vi "phone database.vi"() -> ()   [LabVIEW 2011]
uses:
  <vilib>/addons/database/Auxilliary.llb/DB Tools DataTypes.ctl
  <vilib>/addons/database/Connection.llb/DB Tools Open Connec (Path).vi
  <vilib>/addons/database/NI_Database_API.lvlib
panel:
  out "data":variant[][](array[variant])
  out "column information":T2(array[cluster])
  out "columns":string[](array[string])
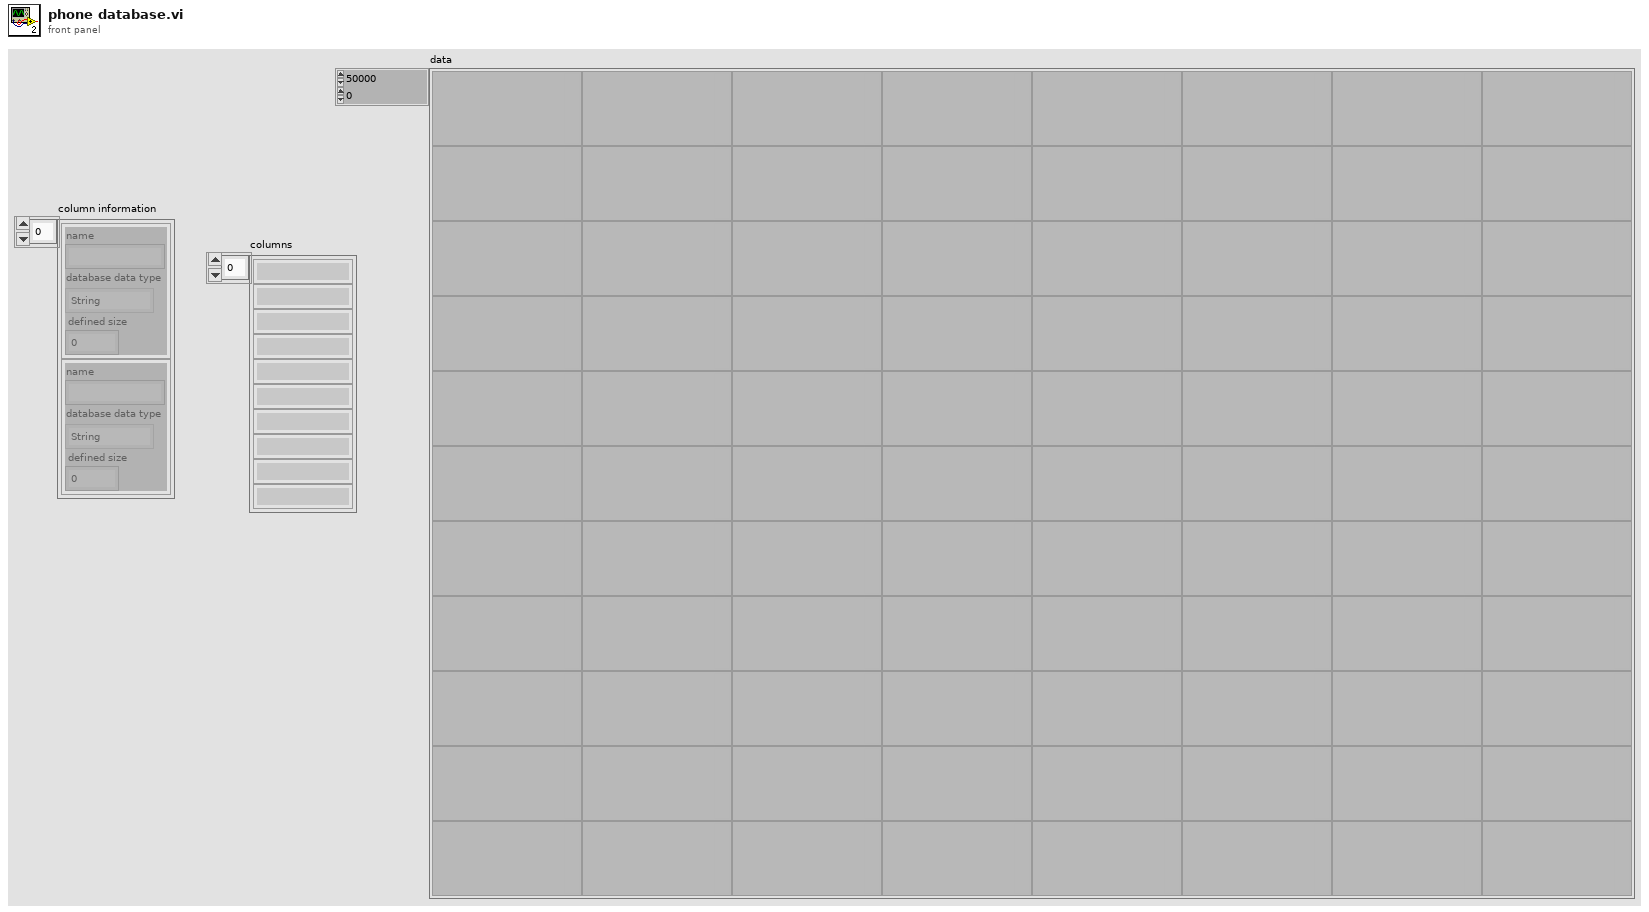
[diagram p1: front panel]
types:
  T1 = typedef "NI_Database_API.lvlib/DB Tools DataTypes.ctl" = enum16{"String", "Long (I32)", "Single (SGL)", "Double (DBL)", "Date/Time", "Binary"}
  T2 = cluster{"name":string, "database data type":T1, "defined size":i32}[]
  T3 = typedef "NI_Database_API.lvlib/Conn ObjectReference.ctl" = refnum<k1>
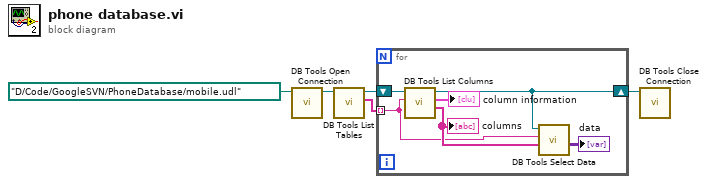
[diagram p0: block diagram]
diagram:
  n1 = call-poly <vilib>:"DB Tools Open Connection.vi"("connection information"=path "D:/Code/GoogleSVN/PhoneDatabase/mobile.udl") -> ("connection reference"=w1:T3)  [unwired: 7 in, 1 out]
  n2 = call <vilib>:"DB Tools List Tables.vi"("connection reference"=w1) -> ("tables"=w4:string[], "connection reference out"=w3:T3)  [unwired: 4 in, 1 out]
  n3 = for {
    tunnel: w4 -> [w7] mode=indexing
    shift-right: [w9] -> w2
    shift-left: w3 -> [w11]
    n4 = call <vilib>:"DB Tools List Columns.vi"("table"=w7, "connection reference"=w11) -> ("columns"=w8:string[], "column information"=→"column information":T2, "connection reference out"=w9:T3)  [unwired: 2 in, 1 out]
    "columns" <- w8
    n5 = call <vilib>:"DB Tools Select Data.vi"("columns"=w8, "table"=w7, "connection reference"=w9) -> ("data"=→"data":variant[][])  [unwired: 3 in, 2 out]
  }
  n6 = call <vilib>:"DB Tools Close Connection.vi"("connection reference"=w2) -> ()  [unwired: 6 in, 1 out]
